vi "FunctionGenerator.vi"(6 "Frequency":dbl caption="FGEN_Frequency", 7 "Waveform Type":enum16{"Sine", "Triangular", "Square"}(ring) caption="FGEN_Waveform_Type", 8 "DC Offset":dbl caption="FGEN_DC_Offset", 9 "Amplitude":dbl caption="FGEN_Amplitude", 10 "Channel":u16(ring) items=["ao0", "ao1"], 11 "Device Name":tag="Dev1") -> (0 "error out":errorcluster, 3 "task out":refnum<k21>)   [LabVIEW 2012]
uses:
  <vilib>/DAQmx/write.llb/DAQmx Write (Analog Wfm 1Chan NSamp).vi
  <vilib>/DAQmx/create/channels.llb/DAQmx Create Channel (AO-Voltage-Basic).vi
  <vilib>/DAQmx/configure/timing.llb/DAQmx Timing (Use Waveform).vi
  <vilib>/DAQmx/miscellaneous.llb/DAQmx Fill In Error Info.vi
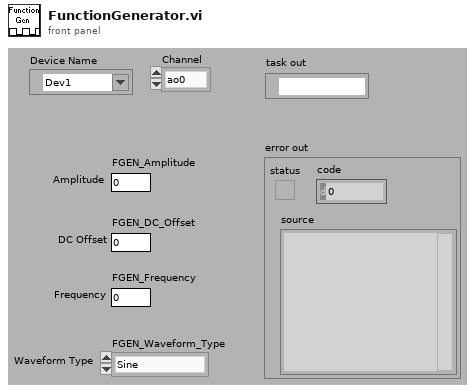
[diagram p1: front panel]
types:
  T1 = enum16{"Sine Wave", "Triangle Wave", "Square Wave", "Sawtooth Wave"}
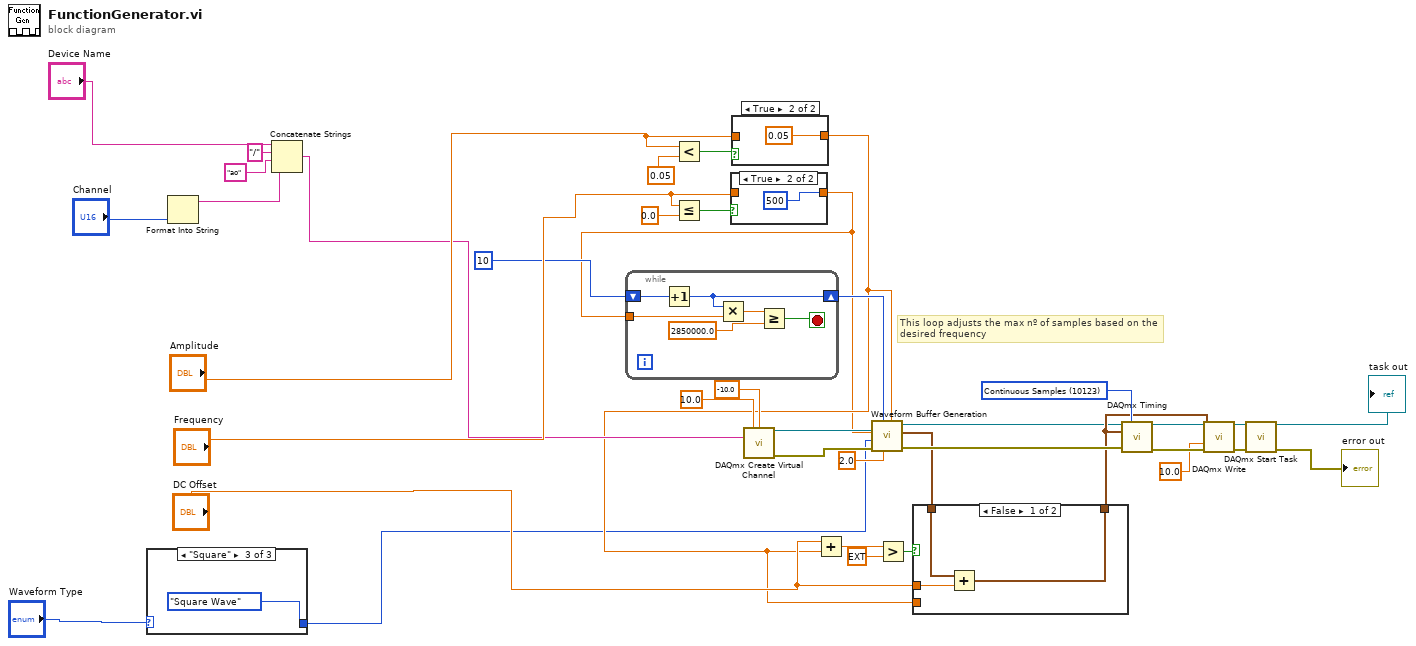
[diagram p0: block diagram]
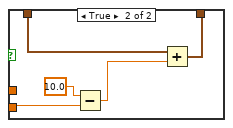
[diagram p4: hidden frame]
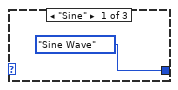
[diagram p5: hidden frame]
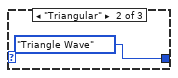
[diagram p6: hidden frame]
diagram:
  w26 = 10123 items=["Finite Samples"=10178, "Continuous Samples"=10123, "Hardware Timed Single Point"=12522] ("sample mode")
  # "This loop adjusts the max nº of samples based on the\ndesired frequency"
  n1 = case shown="\"Square\"" "Waveform Type" {
    tunnel: [T1."Sine Wave" ("Waveform Type") T1."Triangle Wave" ("Waveform Type") T1."Square Wave" ("Waveform Type")] -> w1
    frame "Sine" {
    }
    frame "Triangular" {
    }
    frame "Square" {
    }
  }
  n2 = Format Into String("Channel") -> (resulting string=w32:string)  [unwired: 3 in, 1 out]
  n3 = Concatenate Strings("Device Name", "/" ("string"), "ao" ("string"), w32) -> (w31:string)
  n4 = Less?(x="Amplitude", y=0.05) -> (x < y?=w12:bool)
  n5 = Less Or Equal?(x="Frequency", y=0.0) -> (x <= y?=w10:bool)
  n6 = case shown="True" w10 {
    tunnel: [w43 500] -> w5
    tunnel: "Frequency" -> [w43 _]
    frame False {
    }
    frame True {
    }
  }
  n7 = while {
    shift-right: [w49] -> w8
    shift-left: 10 -> [w50]
    tunnel: w5 -> [w48]
    stop <- w45 stop-if-true
    n8 = Increment(x=w50) -> (x+1=w49:i32)
    n9 = Multiply(x=w49, y=w48) -> (x*y=w47:dbl)
    n10 = Greater Or Equal?(x=w47, y=2850000.0) -> (x >= y?=w45:bool)
  }
  n11 = case shown="True" w12 {
    tunnel: [w51 0.05] -> w7
    tunnel: "Amplitude" -> [w51 _]
    frame False {
    }
    frame True {
    }
  }
  n12 = call-poly <vilib>:"DAQmx Create Virtual Channel.vi"("maximum value"=10.0, "minimum value"=-10.0, "physical channels"=w31) -> ("task out"=w29:refnum<k21>, "error out"=w28:errorcluster)  [unwired: 11 in]
  n13 = Add(x="DC Offset", y=w7) -> (x+y=w17:dbl)
  n14 = call "Waveform Buffer Generation.vi"("Amplitude"=w7, "Cycles per Buffer"=2.0, "Samples per Buffer"=w8, "error in (no error)"=w28, "Waveform Type"=w1, "Desired Frequency"=w5, "task/channels in"=w29) -> ("error out"=w27:errorcluster, "Waveform"=w14:waveform(dbl), "task out"=w4:refnum<k21>)  [unwired: 2 out]
  n15 = Greater?(x=w17, y=ext 10.0) -> (0:w15:bool)
  n16 = case shown="False" w15 {
    tunnel: w14 -> [w55 w60]
    tunnel: w7 -> [_ w57]
    tunnel: "DC Offset" -> [w54 _]
    tunnel: [w53 w59] -> w13
    frame False {
      n17 = Add(x=w55, y=w54) -> (x+y=w53:waveform(dbl))
    }
    frame True {
      n18 = Subtract(x=10.0, y=w57) -> (x-y=w56:dbl)
      n19 = Add(x=w60, y=w56) -> (x+y=w59:waveform(dbl))
    }
  }
  n20 = call-poly <vilib>:"DAQmx Timing.vi"("task/channels in"=w4, "sample mode"=w26, "waveform"=w13, "error in"=w27) -> ("task out"=w25:refnum<k21>, "error out"=w24:errorcluster)  [unwired: 10 in]
  n21 = call-poly <vilib>:"DAQmx Write.vi"("task/channels in"=w25, "data"=w13, "timeout"=10.0, "error in"=w24) -> ("task out"=w22:refnum<k21>, "error out"=w21:errorcluster)  [unwired: 9 in, 1 out]
  n22 = call <vilib>:"DAQmx Start Task.vi"("task/channels in"=w22, "error in"=w21) -> ("task out"=→"task out":refnum<k21>, "error out"=→"error out":errorcluster)  [unwired: 12 in]
